vi "Debug Logger.vi"   [LabVIEW 2009]
uses:
  lib/Apps/App Status Actions.ctl
  lib/Logging/LogFileType.ctl
  lib/Logging/Archive File Type.ctl
types:
  T1 = typedef "App Status Actions.ctl" = enum16{"Init", "Get Status", "Running", "Control", "Autobalanced", "Data Acquisition", "Set App State", "DAQ Started", "Set LBCB State", "Set All", "Set Cont Logging", "Set Step Logging", "Set MM Logging", "Set Volt Logging", "Set DAQ Link"}
  T2 = typedef "LogFileType.ctl" = enum16{"Continuous", "Step", "Volts", "Offsets", "DLL  Errors", "Snapshot", "Commands", "StiffnessUpdates", "Debug", "End List"}
  T3 = typedef "Archive File Type.ctl" = enum16{"LBCB1", "LBCB2", "ExternalSensors", "Combined"}
  T4 = typedef "App Status.ctl" = cluster{"Running":bool, "Controlling L2":bool, "Autobalance L2":bool, "Data Acquisition":bool, " App State":T5, "DAQ Started":bool, "LBCB 1 State":T6, "LBCB 2 State":T6, "Controlling L1":bool, "Autobalance L1":bool, "Continuous Logging":bool, "Step Logging":bool, "Voltage Logging":bool, "Mixed Mode Logging":bool, "DAQ Link":bool}
  T5 = typedef "AppStates.ctl" = enum16{"Starting OM", "Initializing Displays", "Setting up Archiving", "Setting Up DAQ Channels", "Start DAQ", "DAQ Starting", "Controlling LBCBs", "Stopping OM"}
  T6 = typedef "Lbcb Control Loop States.ctl" = enum16{"Idle", "Start Selected", "Load Last Command", "Start Autobalancing", "Autobalancing", "Control Loop Initialized", "Control Enabled"}
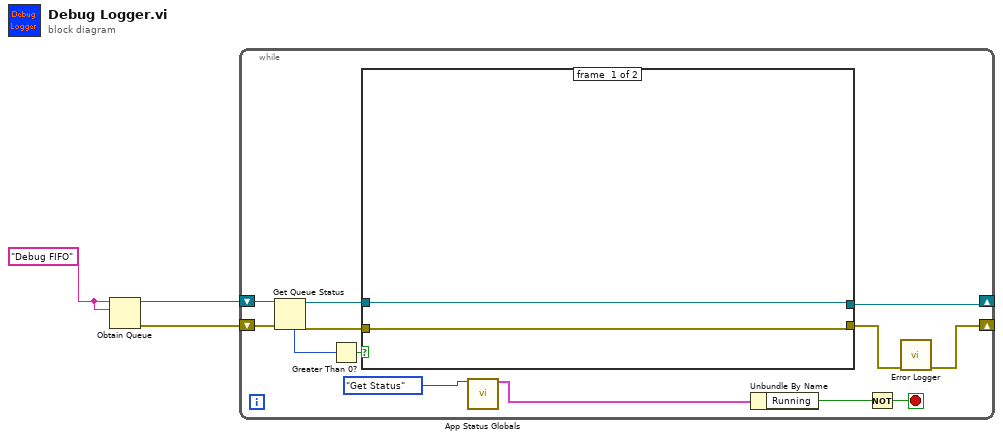
[diagram p0: block diagram]
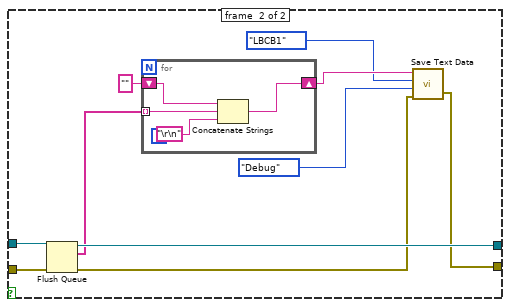
[diagram p2: hidden frame]
diagram:
  w1 = "Debug FIFO" ("name (unnamed)")
  n1 = Obtain Queue(name (unnamed)=w1, element data type=w1) -> (queue out=w3:refnum<queue>, error out=w2:errorcluster)  [unwired: 3 in, 1 out]
  n2 = while {
    shift-right: [w10] -> _
    shift-left: w3 -> [w16]
    shift-right: [w4] -> _
    shift-left: w2 -> [w15]
    stop <- w5 stop-if-true
    n3 = Get Queue Status(queue=w16, error in (no error)=w15) -> (queue out=w12:refnum<queue>, error out=w11:errorcluster, # elements in queue=w13:i32)  [unwired: 1 in, 5 out]
    n4 = Greater Than 0?(x=w13) -> (x > 0?=w14:bool)
    n5 = case shown="True" w14 {
      tunnel: w12 -> [w18 w28]
      tunnel: w11 -> [w17 w27]
      tunnel: [w18 w26] -> w10
      tunnel: [w17 w19] -> w9
      frame #0 {
      }
      frame #1 {
        n6 = Flush Queue(queue=w28, error in (no error)=w27) -> (queue out=w26:refnum<queue>, remaining elements=w25:string[], error out=w20:errorcluster)
        n7 = for {
          tunnel: w25 -> [w32] mode=indexing
          shift-right: [w30] -> w23
          shift-left: "" -> [w29]
          n8 = Concatenate Strings(w29, w32, "\r\n") -> (w30:string)
        }
        n9 = call "Save Text Data.vi"("String"=w23, "Archive File Type"=Archive_File_Type."LBCB1", "LogFile Type"=LogFileType."Debug", "error in"=w20) -> ("error out"=w19:errorcluster)  [unwired: 1 in, 1 out]
      }
    }
    n10 = call "App Status Globals.vi"("App Status Actions"=App_Status_Actions."Get Status") -> ("App Status Out"=w7:T4)  [unwired: 5 in, 9 out]
    n11 = Unbundle By Name(w7) -> ("Running"=w6:bool)
    n12 = Not(x=w6) -> (.not. x?=w5:bool)
    n13 = call "Error Logger.vi"("error in (no error)"=w9) -> ("error out"=w4:errorcluster)  [unwired: 10 in]
  }
